vi "Hilbert.vi"(11 "X":dbl[](array[numeric])) -> (3 "H(X)":dbl[](array[numeric]))   [LabVIEW 2015, in "Digital Signal Processing.lvlib"]
uses:
  Digital Signal Processing.lvlib
  <vilib>/Analysis/NI_AALPro.lvlib
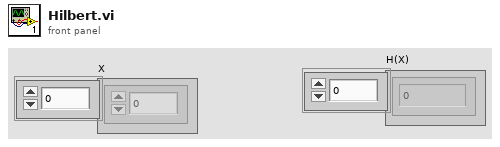
[diagram p1: front panel]
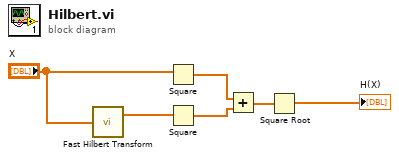
[diagram p0: block diagram]
diagram:
  n1 = call <vilib>:"Fast Hilbert Transform.vi"("X"="X") -> ("Hilbert{X}"=w5:dbl[])  [unwired: 1 out]
  n2 = Square(x="X") -> (x^2=w4:dbl[])
  n3 = Square(x=w5) -> (x^2=w3:dbl[])
  n4 = Add(x=w4, y=w3) -> (x+y=w2:dbl[])
  n5 = Square Root(x=w2) -> (sqrt(x)=→"H(X)":dbl[])
